vi "flow_reg.vi"(0 "SP":dbl caption="setpoint" step=0.01 format="%.2f", 1 "PV":dbl step=0.01 format="%.2f", 2 "Y_H":dbl step=1.0, 3 "controls Y":cluster{"Y_L":dbl, "Y_A":dbl, "Y_D":dbl} {"Y_D" format="%#_13g"; "Y_A" format="%#_13g"; "Y_L" format="%.2f"}, 4 "REG param":T8={"proportional gain (Kc)"=1.0, "integral time (Ti, s)"=10.0, "derivative time (Td, s)"=1.0, "output high"=100.0, "output high start"=40.0, "output high stop"=40.0, "alr value"=0.0, "output low"=0.0, "output rate (EGU/s)"=5.0, "setpoint max"=100.0, "setpoint rate (EGU/min)"=10.0, "stop rate (EGU/min)"=5.0, "deadband"=2.0} {"deadband" min=0.001 format="%.2f"; "setpoint max" format="%.2f"; "stop rate (EGU/min)" min=0.001 format="%.2f"; "setpoint rate (EGU/min)" min=0.001 format="%.2f"; "output high stop" format="%.2f"; "output high start" format="%.2f"; "output rate (EGU/s)" min=0.001 format="%.2f"; "output low" format="%.2f"; "alr value" format="%.2f"; "output high" format="%.2f"; "derivative time (Td, s)" format="%.3f"; "integral time (Ti, s)" format="%.3f"; "proportional gain (Kc)" format="%.3f"}, 6 "Y":T3={"Y_HSw"=1, "Y_HSetState"=enum."auto", "Y_ASetState"=enum."auto", "Y_DSetState"=enum."auto"}, 7 "SP_massiv":dbl[](array[numeric])=[0.0, 10.0, 20.0, 30.0, 40.0, 50.0, 60.0, 70.0, 80.0, 90.0, 100.0] format="%#.2f", 9 "Y_massiv":dbl[](array[numeric])=[0.0, 0.0, 0.0, 0.0, 0.0, 0.0, 0.0, 0.0, 0.0, 0.0, 0.0] format="%#.2f", 10 "Z":cluster{"Z_State":T6, "ZM_State":T7}={"Z_State"=enum."alarm", "ZM_State"=enum."initialization"}, 11 "PV_State":T1, 12 "XB24 (F)":bool) -> (13 "YB":bool, 14 "Y_State":T4={"Y_Source"=enum."local disabled", "Y_SetState"=enum."auto", "SP_Set"=0.0, "SP"=0.0, "PV"=0.0, "Y"=0.0, "Y_State"={"code"=0, "visible"=FALSE, "color"=0, "source"=""}, "YB"=FALSE} {"SP" step=0.01 format="%.2f"; "Y" format="%.2f"; "PV" format="%.2f"; "SP_Set" step=0.01 format="%.2f"}, 15 "Y":dbl format="%.2f", 17 "T":u32, 18 "End":bool)   [LabVIEW 2019, in "control.lvlib"]
uses:
  control.lvlib
  Heating/ctl/Z_State.ctl
  Heating/ctl/ZM_State.ctl
  Heating/ctl/Y.ctl
  Heating/ctl/Y_source.ctl
  Heating/ctl/Y_state.ctl
  Inputs/Ctl/Parameter State.ctl
  PID/PID Output Rate Limiter.vi
  PID/PID Timing Estimation.vi
  Trigers/D^.vi
  Timer Delay/Timer.vi
  PID/PID Output Rate Limiter Ext.vi
  PID/PID Timing Estimation Ext.vi
  Inputs/Sensor 2P.vi
  Heating/Heating.lvlib
  Userlib.lvlib
  Counter/Counter.lvlib
  Logik/Logik.lvlib
  Inputs/Inputs.lvlib
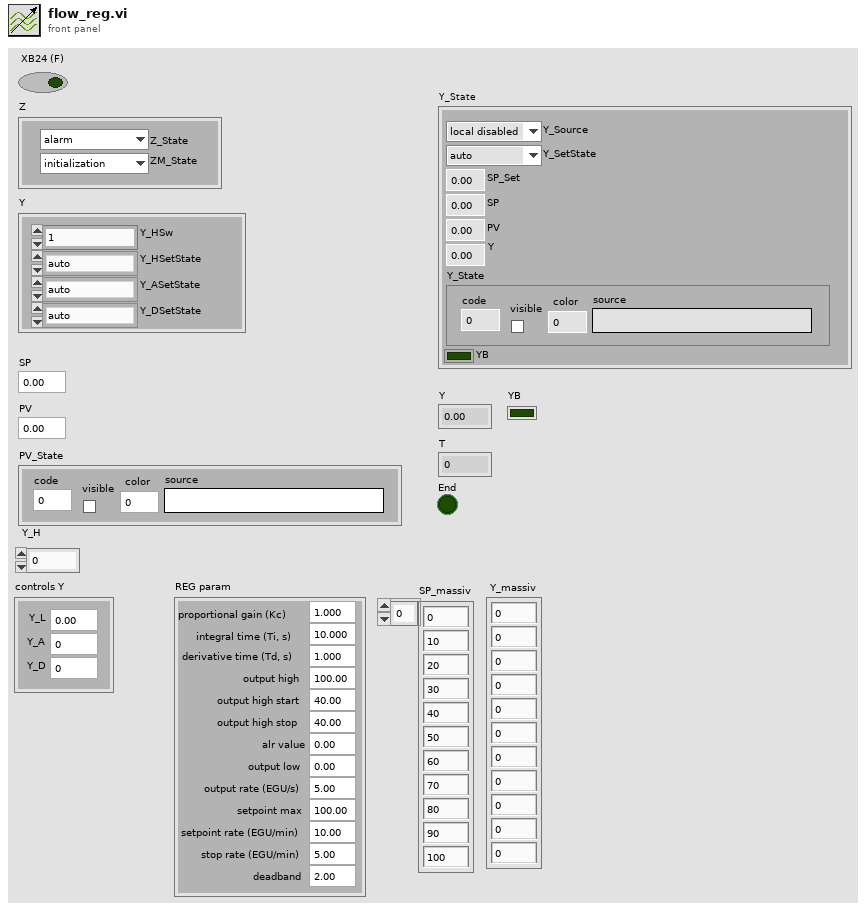
[diagram p1: front panel]
types:
  T1 = typedef "Inputs.lvlib/Parameter State.ctl" = cluster{"code":i32, "visible":bool, "color":u32, "source":string}
  T2 = typedef "Heating.lvlib/Y_state.ctl" = enum8{"initialize", "alarm", "min", "stop", "hand", "auto", "max"}
  T3 = cluster{"Y_HSw":u32, "Y_HSetState":T2, "Y_ASetState":T2, "Y_DSetState":T2}
  T4 = typedef "Heating.lvlib/Y.ctl" = cluster{"Y_Source":T5, "Y_SetState":T2, "SP_Set":dbl, "SP":dbl, "PV":dbl, "Y":dbl, "Y_State":T1, "YB":bool}
  T5 = typedef "Heating.lvlib/Y_source.ctl" = enum8{"initialize", "local disabled", "local hand", "hand", "auto", "dist"}
  T6 = typedef "Heating.lvlib/Z_State.ctl" = enum8{"initialization", "alarm", "disabled", "not ready", "stop ready", "reserv", "switched off", "reserv2", "switched on", "check", "on min", "decrease out", "on", "increase out", "on max"}
  T7 = typedef "Heating.lvlib/ZM_State.ctl" = enum8{"initialization", "stop", "start_cmd", "contactor_on_cmd", "heating", "on", "stop_cmd", "power_down", "contactor_off_cmd", "cooling", "restart_delay"}
  T8 = cluster{"proportional gain (Kc)":dbl, "integral time (Ti, s)":dbl, "derivative time (Td, s)":dbl, "output high":dbl, "output high start":dbl, "output high stop":dbl, "alr value":dbl, "output low":dbl, "output rate (EGU/s)":dbl, "setpoint max":dbl, "setpoint rate (EGU/min)":dbl, "stop rate (EGU/min)":dbl, "deadband":dbl}
  T9 = cluster{"proportional gain (Kc)":dbl, "integral time (Ti, s)":dbl, "derivative time (Td, s)":dbl, "output high":dbl, "output high start":dbl, "output high stop":dbl, "alr value":dbl, "output low":dbl, "output rate (EGU/s)":dbl, "setpoint max":dbl, "setpoint rate (EGU/min)":dbl, "stop rate (EGU/min)":dbl}
  T10 = typedef "control.lvlib/PID param.ctl" = cluster{"proportional gain (Kc)":dbl, "integral time (Ti, s)":dbl, "derivative time (Td, s)":dbl, "output high":dbl, "alr value":dbl, "output low":dbl, "output rate (EGU/s)":dbl, "dt (s)":dbl}
  T11 = enum8{"alarm", "min", "stop", "hand", "auto", "max"}
  T12 = cluster{"Y_Source":T5, "Y_SetState":T2, "SP":dbl, "output":dbl, "PV":dbl, "output":dbl, "PV_State":T1, bool}
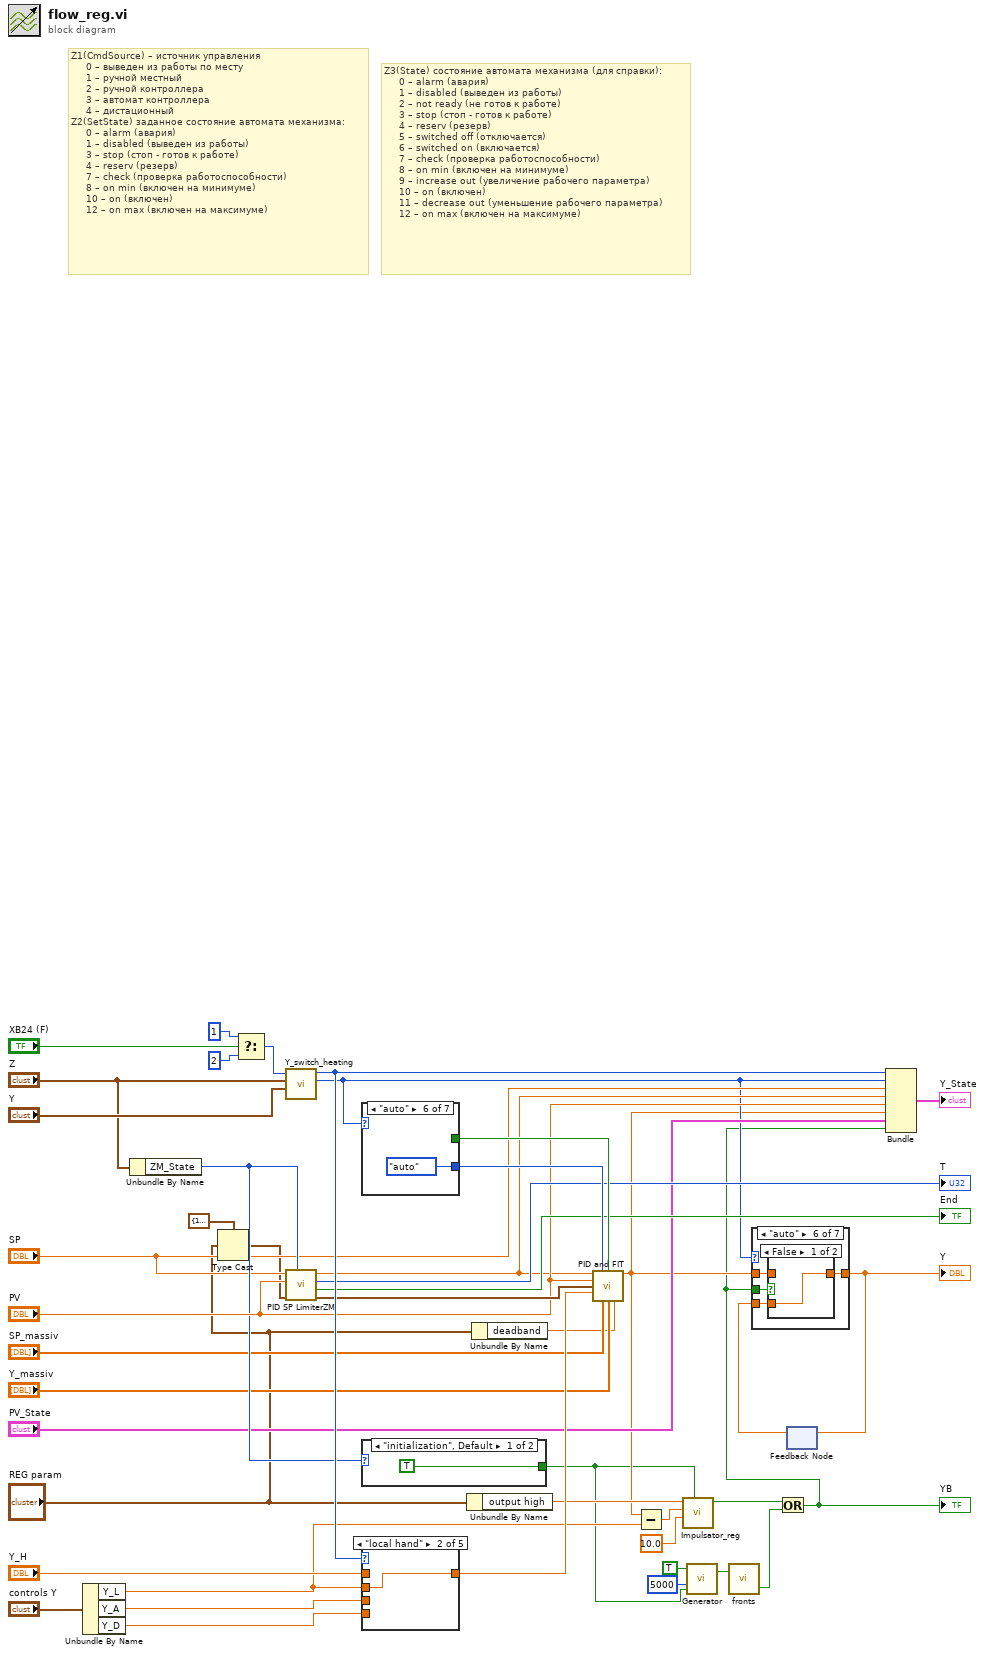
[diagram p0: block diagram]
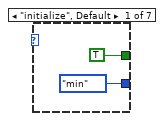
[diagram p9: hidden frame]
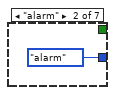
[diagram p10: hidden frame]
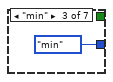
[diagram p11: hidden frame]
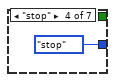
[diagram p12: hidden frame]
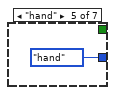
[diagram p13: hidden frame]
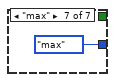
[diagram p14: hidden frame]
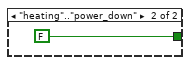
[diagram p15: hidden frame]
diagram:
  # "Z1(CmdSource) – источник управления\n     0 – выведен из работы по месту\n     1 – ручной местный\n     2 – ручной контроллера\n     3 – автомат контроллера\n     4 – дистационный\nZ2(SetState) заданное состояние автомата механизма:\n     0 – alarm (авария)\n     1 – disabled (выведен из работы)\n     3 – stop (стоп - готов к работе)\n     4 – reserv (резерв)\n     7 – check (проверка работоспособности)\n     8 – on min (включен на минимуме)\n     10 – on (включен)\n     12 – on max (включен на максимуме)"
  # "Z3(State) состояние автомата механизма (для справки):\n     0 – alarm (авария)\n     1 – disabled (выведен из работы)\n     2 – not ready (не готов к работе)\n     3 – stop (стоп - готов к работе)\n     4 – reserv (резерв)\n     5 – switched off (отключается)\n     6 – switched on (включается)\n     7 – check (проверка работоспособности)\n     8 – on min (включен на минимуме)\n     9 – increase out (увеличение рабочего параметра)\n     10 – on (включен)\n     11 – decrease out (уменьшение рабочего параметра)\n     12 – on max (включен на максимуме)"
  n1 = Unbundle By Name("controls Y") -> ("Y_L"=w19:dbl, "Y_A"=w43:dbl, "Y_D"=w42:dbl)
  n2 = Unbundle By Name("Z") -> ("ZM_State"=w26:T7)
  n3 = Type Cast(type=T9 {"proportional gain (Kc)"=1.0, "integral time (Ti, s)"=10.0, "derivative time (Td, s)"=1.0, "output high"=100.0, "output high start"=40.0, "output high stop"=40.0, "alr value"=0.0, "output low"=0.0, "output rate (EGU/s)"=5.0, "setpoint max"=100.0, "setpoint rate (EGU/min)"=10.0, "stop rate (EGU/min)"=5.0} ("REG param"), x="REG param") -> (*(type *) &x=w2:T9)
  n4 = Select(t=u32 1, s="XB24 (F)", f=u32 2 ("Y_HSw")) -> (s? t:f=w37:u32)
  n5 = call "Y_switch_heating.vi"("Y"="Y", "Z"="Z", "Y_LSw (2-auto)"=w37) -> ("Y_SetState"=w21:T2, "Y_Source"=w35:T5)  [unwired: 7 in]
  n6 = call "PID SP LimiterZM.vi"("ZM_State"=w26, "REG param"=w2, "PV"="PV", "SP"="SP") -> ("PID param"=w31:T10, "End"=→"End":bool, "T"=→"T":u32, "output"=w25:dbl)  [unwired: 4 in]
  n7 = case shown="\"auto\"" w21 {
    tunnel: [T11."min" ("X1(SetState)") T11."alarm" ("X1(SetState)") T11."min" ("X1(SetState)") T11."stop" ("X1(SetState)") T11."hand" ("X1(SetState)") T11."auto" ("X1(SetState)") T11."max" ("X1(SetState)")] -> w33
    tunnel: [TRUE _ _ _ _ _ _] -> w32
    frame "initialize", Default {
    }
    frame "alarm" {
    }
    frame "min" {
    }
    frame "stop" {
    }
    frame "hand" {
    }
    frame "auto" {
    }
    frame "max" {
    }
  }
  n8 = case shown="\"initialization\", Default" w26 {
    tunnel: [TRUE FALSE] -> w11
    frame "initialization", Default {
    }
    frame "heating".."power_down" {
    }
  }
  n9 = case shown="\"local hand\"" w35 {
    tunnel: "Y_H" -> [_ _ w57 _ _]
    tunnel: w19 -> [w55 w56 _ _ _]
    tunnel: w42 -> [_ _ _ _ w59]
    tunnel: [w55 w56 w57 w58 w59] -> w40
    tunnel: w43 -> [_ _ _ w58 _]
    frame "local disabled", Default {
    }
    frame "local hand" {
    }
    frame "hand" {
    }
    frame "auto" {
    }
    frame "dist" {
    }
  }
  n10 = Unbundle By Name("REG param") -> ("output high"=w17:dbl)
  n11 = Unbundle By Name("REG param") -> ("deadband"=w1:dbl)
  n12 = call "PID and FIT.vi"("setpoint"=w25, "X1(SetState)"=w33, "reinitialize? (F)"=w32, "process variable"="PV", "PID param"=w31, "manual control"=w40, "SP_massiv"="SP_massiv", "Y_massiv"="Y_massiv", "deadband"=w1) -> ("output"=w14:dbl)  [unwired: 5 in, 1 out]
  n13 = Subtract(x=w14, y=w19) -> (x-y=w16:dbl)
  n14 = call "Impulsator_reg.vi"("Initialise"=w11, "proportional gain (Kc)"=10.0, "PV"=w16, "upper limit"=w17) -> ("Y"=w6:bool)  [unwired: 7 in]
  n15 = call "Generator.vi"("R"=w11, "T ms (500)"=5000, "ON (F)"=TRUE) -> ("Q"=w10:bool)  [unwired: 1 in]
  n16 = call "fronts.vi"("in"=w10) -> ("fall"=w9:bool)  [unwired: 1 in, 1 out]
  n17 = Or(x=w6, y=w9) -> (x .or. y?=w5:bool)
  "YB" <- w5
  n18 = feedback #1() -> (w20:dbl)  [unwired: 1 in]
  n19 = case shown="\"auto\"" w21 {
    tunnel: w14 -> [w60 w61 w62 w63 w64 w66 w71]
    tunnel: [w60 w61 w62 w63 w64 w67 w71] -> w18
    tunnel: w20 -> [_ _ _ _ _ w65 _]
    tunnel: w5 -> [_ _ _ _ _ w68 _]
    frame "initialize", Default {
    }
    frame "alarm" {
    }
    frame "min" {
    }
    frame "stop" {
    }
    frame "hand" {
    }
    frame "auto" {
      n20 = case shown="False" w68 {
        tunnel: [w69 w70] -> w67
        tunnel: w66 -> [_ w70]
        tunnel: w65 -> [w69 _]
        frame False {
        }
        frame True {
        }
      }
    }
    frame "max" {
    }
  }
  "Y" <- w18
  n21 = feedback-in #1(w18) -> ()
  n22 = Bundle("Y_Source"=w35, "Y_SetState"=w21, "SP"="SP", "output"=w25, "PV"="PV", "output"=w14, "PV_State"="PV_State", w5) -> (→"Y_State":T12)  [unwired: 1 in]
